vi "Data Server.vi"() -> ()   [LabVIEW 2012]
doc: "Date Server.vi sends the current time and date via TCP to all Date Client.vi's that connect to it. It is composed of two parts: first, a loop that listens for each client to connect; and second, a loop that send the date and time to each connection in the queue."
uses:
  command cluster.ctl
  command.ctl
  Server stats.ctl
  Dataserver method.ctl
  data w time.ctl
panel:
  in  "Save method":bool
  in  "Load method":bool
  in  "Tab Control":enum32{"Stats", "Server Method", "Errors"}(tab)=enum."Server Method"
  out "data out":T1 {"seconds since 1904" format="%<%I:%M:%S %p\n%m/%d/%Y>T"; "voltage data" format="%.4f"}
  out "recent data loss time":dbl format="%<%I:%M:%S %p\n%m/%d/%Y>T"
  out "lost data":bool
  in  "max buffer":i32=1000
  out "scan rate (Hz)":dbl format="%.2f"
  out "time at AI start":dbl format="%<%I:%M:%S %p\n%m/%d/%Y>T"
  in  "update states":u32=50
  out "local buffer size":i32
  in  "write Server stats":i32=5000
  out "total  logons":i32
  out "scans backlog":u32
  out "Server Stats":T2={"scan rate"=10.0, "# connections"=0, "channel settings"=[]} {"channel settings"."lower input limits" format="%.4f"; "channel settings"."upper input limits" format="%.4f"; "scan rate" format="%.2f"}
  in  "write data":i32=5000 min=1 max=30000 step=1
  in  "read states":i32=5000 min=1 max=30000 step=1
  out "state array":T3[](array[typedef]) {"Scans per Sample" min=1}
  out "connections":i32
  in  "Server Method":T5={"scan rate (Hz)"=500.0, "Channel group array"=[{"channels"="SC1Mod1/ai0", "max voltage"=0.02, "Port locations"="what"}, {"channels"="SC1Mod1/ai0", "max voltage"=10.0, "Port locations"=""}, {"channels"="SC1Mod1/ai1:7", "max voltage"=1.0, "Port locations"="next"}, {"channels"="SC1Mod1/ai8:11", "max voltage"=10.0, "Port locations"="final"}, {"channels"="SC1Mod1/ai12:15", "max voltage"=0.01, "Port locations"="finaler"}, {"channels"="SC1Mod1/ai16:31", "max voltage"=0.5, "Port locations"="finalist"}, {"channels"="SC1Mod2/ai0:31", "max voltage"=0.1, "Port locations"="last"}], "Number of groups"=7} {"Number of groups" min=1; "Channel group array"."max voltage" format="%.4f"; "scan rate (Hz)" format="%.2f"}
  out "listen halted":bool=TRUE
  out "Quit all":bool
  out "default dsm":refnum<file>
  out "TCP error":errorcluster
  out "DAQ error":errorcluster
  out "listen loop error":errorcluster
  in  "port":u16=6341
  out "listener ID":refnum<k5>
  out "taskID":refnum<k21>
  in  "Apply Method":bool
  in  "Quit":bool
  out "connections":refnum<k5>[](array[refnum])
  # "timing (ms)"
  # "ms"
  # "ms"
  # "ms"
  # "ms"
  # "Hz"
  # "Hz"
  # "channel identifiers"
  # "max voltage"
  # "port locations"
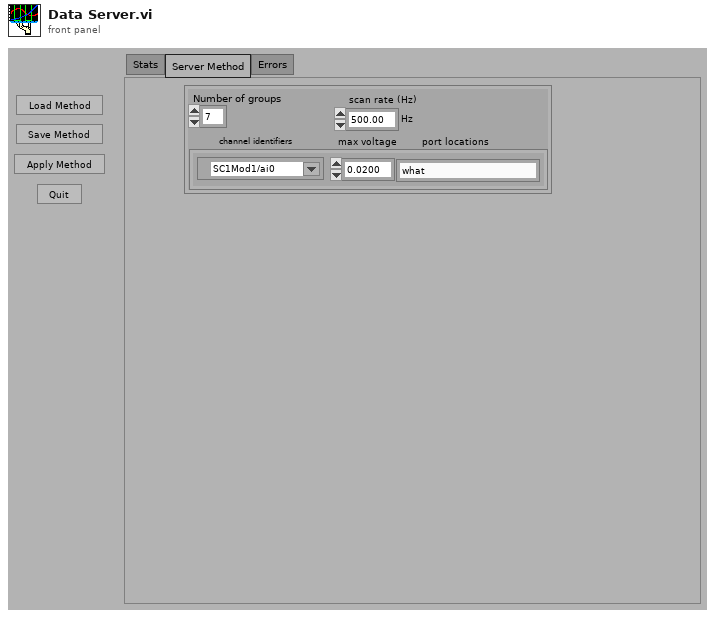
[diagram p1: front panel]
types:
  T1 = typedef "data w time.ctl" = cluster{"voltage data":sgl[], "seconds since 1904":dbl, "arbtrary scans":u32}
  T2 = typedef "Server stats.ctl" = cluster{"scan rate":dbl, "# connections":i32, "channel settings":cluster{"Name":string, "upper input limits":sgl, "lower input limits":sgl, "Location":string}[]}
  T3 = typedef "command cluster.ctl" = cluster{"command":T4, "start time (ms)":u32, "Channel Indices":i32[], "Scans per Sample":i32}
  T4 = typedef "command.ctl" = enum16{"Idle", "Send Data", "Send 1 Scan", "Logoff"}
  T5 = typedef "Dataserver method.ctl" = cluster{"scan rate (Hz)":dbl, "Channel group array":cluster{"channels":tag, "max voltage":sgl, "Port locations":string}[], "Number of groups":u8}
  T6 = enum16{"clear", "add connection", "change command", "write state", "delete connection", "read"}
  T7 = enum16{"open", "open or create", "create or replace", "create", "open (read only)"}
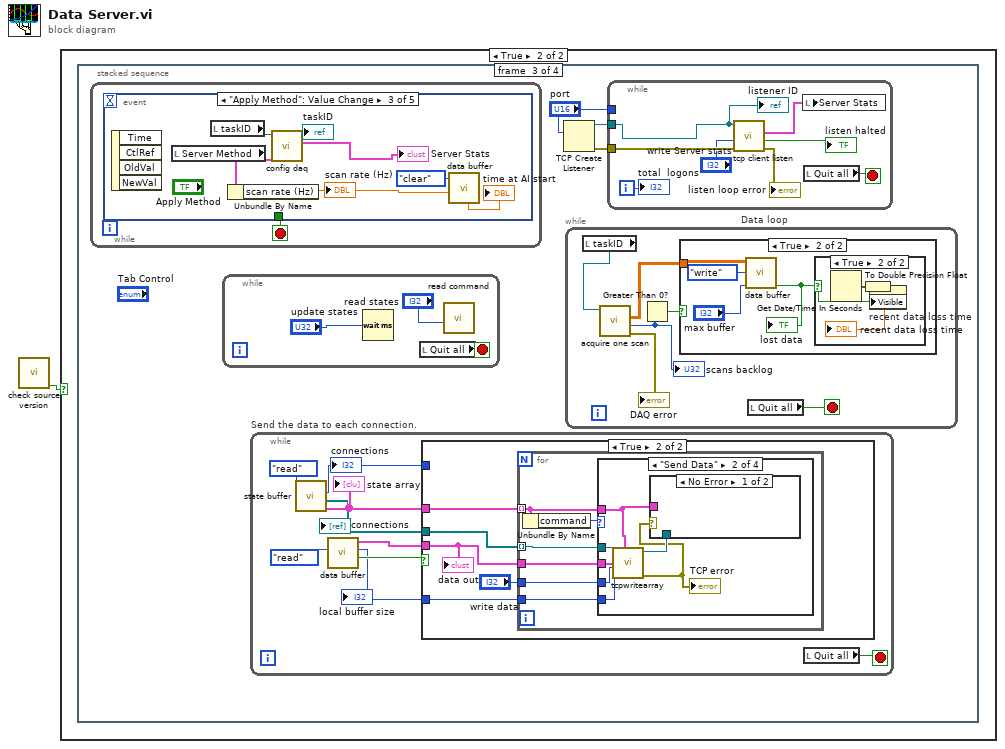
[diagram p0: block diagram]
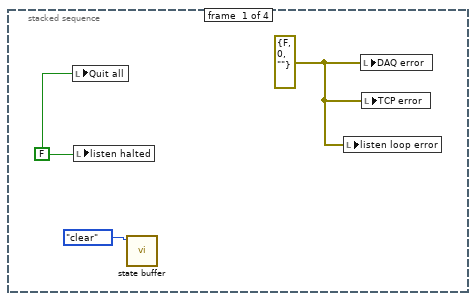
[diagram p3: hidden frame]
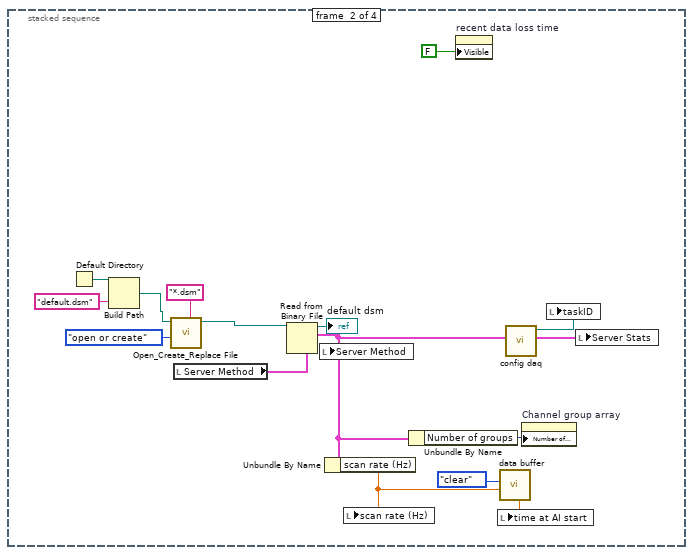
[diagram p4: hidden frame]
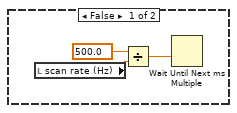
[diagram p7: hidden frame]
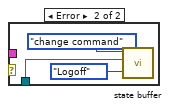
[diagram p9: hidden frame]
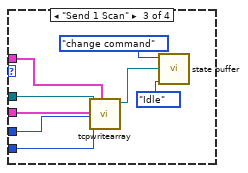
[diagram p10: hidden frame]
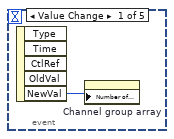
[diagram p12: hidden frame]
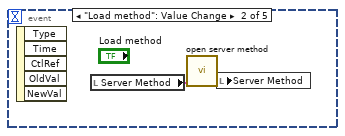
[diagram p13: hidden frame]
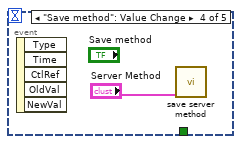
[diagram p14: hidden frame]
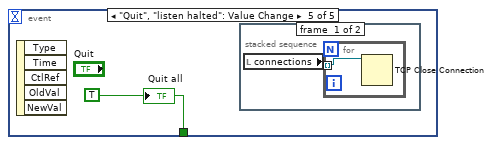
[diagram p15: hidden frame]
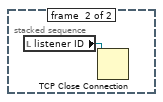
[diagram p16: hidden frame]
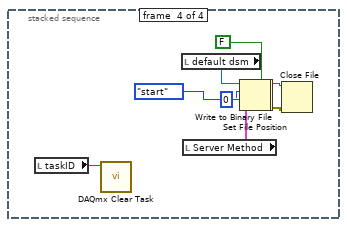
[diagram p17: hidden frame]
diagram:
  n1 = call "check source version.vi"() -> ("continue running?"=w1:bool)  [unwired: 2 in, 3 out]
  n2 = case shown="True" w1 {
    frame False {
    }
    frame True {
      n3 = stacked-sequence {
        frame #0 {
          w3 = errorcluster {"status"=FALSE, "code"=0, "source"=""} ("DAQ error")
          w4 = FALSE ("Write Attribute")
          n4 = local write "Quit all"(w4) -> ()
          n5 = local write "listen halted"(w4) -> ()
          n6 = call "state buffer.vi"("command"=T6."clear") -> ()  [unwired: 8 in, 3 out]
          n7 = local write "listen loop error"(w3) -> ()
          n8 = local write "DAQ error"(w3) -> ()
          n9 = local write "TCP error"(w3) -> ()
        }
        frame #1 {
          n10 = Default Directory() -> (w17:path)
          n11 = Build Path(base path=w17, name or relative path="default.dsm") -> (appended path=w16:path)
          n12 = call <vilib>:"Open_Create_Replace File.vi"("pattern"="*.dsm", "function (open:0)"=T7."open or create", "file path"=w16) -> ("refnum"=w19:refnum<file>)  [unwired: 5 in, 3 out]
          n13 = local read "Server Method"() -> (w18:T5)
          n14 = Read from Binary File(5:w18, 11:w19) -> (2:w10:T5, 3:→"default dsm":refnum<file>)  [unwired: 4 in, 2 out]
          n15 = local write "Server Method"(w10) -> ()
          n16 = Unbundle By Name(w10) -> ("scan rate (Hz)"=w6:dbl)
          n17 = local write "scan rate (Hz)"(w6) -> ()
          n18 = Unbundle By Name(w10) -> ("Number of groups"=w9:u8)
          n19 = property on="recent data loss time" class="DigNum (strict)"("Visible"=FALSE) -> ()  [unwired: 2 in, 2 out]
          n20 = call "data buffer.vi"("action"=enum16{"write", "read", "clear"}."clear", "scan rate (Hz)"=w6) -> ("time at AI start"=w7:dbl)  [unwired: 2 in, 5 out]
          n21 = local write "time at AI start"(w7) -> ()
          n22 = call "config daq.vi"("Server Method"=w10) -> ("task out"=w12:refnum<k21>, "Server Stats"=w11:T2)  [unwired: 8 in]
          n23 = property on="Channel group array" class="Arr (strict)"("Number of Rows"=w9) -> ()  [unwired: 2 in, 2 out]
          n24 = local write "taskID"(w12) -> ()
          n25 = local write "Server Stats"(w11) -> ()
        }
        frame #2 {
          n26 = while {
            stop <- w89 stop-if-true
            n27 = event shown="[2] \"Apply Method\": Value Change" {
              selector: _ -> [_ _ _ _ _]
              dyn-events: _ -> [_ _ _ _ _]
              timeout: _ -> [_ _ _ _ _]
              tunnel: [_ _ _ _ w101] -> w89
              event Value Change {
                n28 = event-data() -> ("NewVal"=w90:u8)  [unwired: 1 in, 4 out]
                n29 = property on="Channel group array" class="Arr (strict)"("Number of Rows"=w90) -> ()  [unwired: 2 in, 2 out]
              }
              event "Load method": Value Change {
                n30 = event-data() -> ()  [unwired: 1 in, 5 out]
                n31 = local read "Server Method"() -> (w92:T5)
                n32 = call "open server method.vi"("DS method in"=w92) -> ("DS method"=w91:T5)  [unwired: 8 in, 1 out]
                n33 = local write "Server Method"(w91) -> ()
              }
              event "Apply Method": Value Change {
                n34 = event-data() -> ()  [unwired: 1 in, 4 out]
                n35 = local read "Server Method"() -> (w99:T5)
                n36 = local read "taskID"() -> (w97:refnum<k21>)
                n37 = Unbundle By Name(w99) -> ("scan rate (Hz)"=w95:dbl)
                "scan rate (Hz)" <- w95
                n38 = call "config daq.vi"("task in"=w97, "Server Method"=w99) -> ("task out"=→"taskID":refnum<k21>, "Server Stats"=→"Server Stats":T2)  [unwired: 7 in]
                n39 = call "data buffer.vi"("action"=enum16{"write", "read", "clear"}."clear", "scan rate (Hz)"=w95) -> ("time at AI start"=→"time at AI start":dbl)  [unwired: 2 in, 5 out]
              }
              event "Save method": Value Change {
                n40 = event-data() -> ()  [unwired: 1 in, 5 out]
                n41 = call "save server method.vi"("DS method"="Server Method") -> ()  [unwired: 10 in]
              }
              event "Quit", "listen halted": Value Change {
                w101 = TRUE ("Quit all")
                n42 = event-data() -> ()  [unwired: 1 in, 5 out]
                n43 = stacked-sequence {
                  frame #0 {
                    n44 = local read "connections"() -> (w102:refnum<k5>[])
                    n45 = for {
                      tunnel: w102 -> [w103] mode=indexing
                      n46 = TCP Close Connection(connection ID=w103) -> ()  [unwired: 2 in, 2 out]
                    }
                  }
                  frame #1 {
                    n47 = local read "listener ID"() -> (w104:refnum<k5>)
                    n48 = TCP Close Connection(connection ID=w104) -> ()  [unwired: 2 in, 2 out]
                  }
                }
                "Quit all" <- w101
              }
            }
          }
          n49 = while {
            stop <- w26 stop-if-true
            n50 = Wait (ms)(milliseconds to wait="update states") -> ()  [unwired: 1 out]
            n51 = local read "Quit all"() -> (w26:bool)
            n52 = call "read command.vi"("timeout ms (25000)"="read states") -> ()  [unwired: 8 in, 3 out]
          }
          n53 = while "Send the data to each connection." {
            stop <- w48 stop-if-true
            n54 = call "state buffer.vi"("command"=T6."read") -> ("state array"=w43:T3[], "connections"=w42:refnum<k5>[], "clients"=w40:i32)  [unwired: 8 in]
            "connections" <- w42
            "state array" <- w43
            "connections" <- w40
            n55 = call "data buffer.vi"("action"=enum16{"write", "read", "clear"}."read") -> ("data out"=w47:T1, "buffer size"=w44:i32, "got data"=w45:bool)  [unwired: 3 in, 3 out]
            "local buffer size" <- w44
            n56 = case shown="True" w45 {
              tunnel: w47 -> [_ w55]
              tunnel: w42 -> [_ w54]
              tunnel: w43 -> [_ w53]
              tunnel: w40 -> [_ _]
              tunnel: w44 -> [_ w52]
              frame False {
                n57 = local read "scan rate (Hz)"() -> (w49:dbl)
                n58 = Divide(x=500.0, y=w49) -> (x/y=w50:dbl)
                n59 = Wait Until Next ms Multiple(millisecond multiple=w50) -> ()  [unwired: 1 out]
              }
              frame True {
                n60 = for {
                  tunnel: w53 -> [w61] mode=indexing
                  tunnel: w54 -> [w62] mode=indexing
                  tunnel: "write data" -> [w60]
                  tunnel: w55 -> [w58]
                  tunnel: w52 -> [w57]
                  n61 = Unbundle By Name(w61) -> ("command"=w59:T4)
                  n62 = case shown="\"Send Data\"" w59 {
                    tunnel: w62 -> [_ w69 w80 _]
                    tunnel: w61 -> [_ w68 w77 _]
                    tunnel: w60 -> [_ w63 w79 _]
                    tunnel: w58 -> [_ w67 w78 _]
                    tunnel: w57 -> [_ w65 w73 _]
                    frame .."Idle" {
                    }
                    frame "Send Data" {
                      n63 = call "tcpwritearray.vi"("command cluster"=w68, "buffer size"=w65, "timeout ms (25000)"=w63, "data"=w67, "refnum in"=w69) -> ("error out"=w64:errorcluster, "refnum out"=w66:refnum<k5>)  [unwired: 4 in, 1 out]
                      "TCP error" <- w64
                      n64 = case shown="No Error" w64 {
                        tunnel: w68 -> [_ _]
                        tunnel: w66 -> [_ w71]
                        frame No Error {
                        }
                        frame Error {
                          n65 = call "state buffer.vi"("change command"=command."Logoff", "connection"=w71, "command"=T6."change command") -> ()  [unwired: 6 in, 3 out]
                        }
                      }
                    }
                    frame "Send 1 Scan" {
                      n66 = call "tcpwritearray.vi"("command cluster"=w77, "buffer size"=w73, "timeout ms (25000)"=w79, "data"=w78, "refnum in"=w80) -> ("refnum out"=w75:refnum<k5>)  [unwired: 4 in, 2 out]
                      n67 = call "state buffer.vi"("change command"=command."Idle", "connection"=w75, "command"=T6."change command") -> ()  [unwired: 6 in, 3 out]
                    }
                    frame "Logoff" {
                      # "this will only happen if\ntwo clients logoff\nin the same iteration"
                    }
                  }
                }
                "data out" <- w55
              }
            }
            n68 = local read "Quit all"() -> (w48:bool)
          }
          n69 = TCP Create Listener(10:"port") -> (0:w22:errorcluster, 3:w23:refnum<k5>)  [unwired: 4 in, 1 out]
          n70 = while "Data loop" {
            stop <- w32 stop-if-true
            n71 = local read "taskID"() -> (w28:refnum<k21>)
            n72 = call "acquire one scan.vi"("taskID in"=w28) -> ("error out"=→"DAQ error":errorcluster, "scans read"=w30:u32, "voltage data"=w27:dbl[][])  [unwired: 6 in, 2 out]
            "scans backlog" <- w30
            n73 = Greater Than 0?(x=w30) -> (x > 0?=w29:bool)
            n74 = case shown="True" w29 {
              tunnel: w27 -> [_ w36]
              frame False {
              }
              frame True {
                n75 = call "data buffer.vi"("voltage data"=w36, "action"=enum16{"write", "read", "clear"}."write", "max buffer"="max buffer") -> ("lost data"=w33:bool)  [unwired: 1 in, 5 out]
                "lost data" <- w33
                n76 = case shown="True" w33 {
                  selector: w33 -> [_ w38]
                  frame False {
                  }
                  frame True {
                    n77 = Get Date/Time In Seconds() -> (seconds since 1Jan1904=w37:timestamp)
                    n78 = To Double Precision Float(number=w37) -> (double precision float=→"recent data loss time":dbl)
                    n79 = property on="recent data loss time" class="DigNum (strict)"("Visible"=w38) -> ()  [unwired: 2 in, 2 out]
                  }
                }
              }
            }
            n80 = local read "Quit all"() -> (w32:bool)
          }
          n81 = while {
            tunnel: w22 -> [w88]
            tunnel: w23 -> [w81]
            tunnel: "port" -> [_]
            i -> [w84]
            stop <- w85 stop-if-true
            n82 = call "tcp client listen.vi"("error in (no error)"=w88, "write Server stats timeout"="write Server stats", "listener ID in"=w81) -> ("listen loop error out"=→"listen loop error":errorcluster, "listen halted"=→"listen halted":bool, "Server Stats out"=w82:T2)  [unwired: 6 in]
            n83 = local write "Server Stats"(w82) -> ()
            n84 = local read "Quit all"() -> (w85:bool)
            "listener ID" <- w81
            "total  logons" <- w84
          }
        }
        frame #3 {
          n85 = local read "taskID"() -> (w105:refnum<k21>)
          n86 = call <vilib>:"DAQmx Clear Task.vi"("task in"=w105) -> ()  [unwired: 14 in, 1 out]
          n87 = local read "default dsm"() -> (w114:refnum<file>)
          n88 = local read "Server Method"() -> (w111:T5)
          n89 = Set File Position(offset (in bytes) (0)=0 ("pos offset (0)"), refnum=w114, from (0:start)=enum16{"start", "end", "current"}."start" ("pos mode (0:2)")) -> (refnum out=w108:refnum<file>, error out=w107:errorcluster)  [unwired: 1 in]
          n90 = Write to Binary File(file (use dialog)=w108, data=w111, error in=w107, 5:FALSE ("prepend array or string size? (T)")) -> (refnum out=w112:refnum<file>, error out=w113:errorcluster)  [unwired: 2 in, 1 out]
          n91 = Close File(refnum=w112, error in=w113) -> ()  [unwired: 2 out]
        }
      }
    }
  }
